vi "Gunner.vi"(8 "error in (no error)":errorcluster, 10 "Map":i32[](array[numeric]), 11 "Gunner In":refnum<class "Cross.lvclass">) -> (0 "error out":errorcluster, 1 "Direction":T1, 2 "Action":T2, 3 "Gunner Out":refnum<class "Cross.lvclass">, 4 "Replicated Class":refnum<class "Cross.lvclass">)   [LabVIEW 2015, in "Cross.lvclass"]
uses:
  Cross.lvclass
  Type Defs/Action Enum.ctl
  Type Defs/Direction Enum.ctl
  Cross.lvclass/Cross.ctl
  Type Defs/SB Type Defs.lvlib
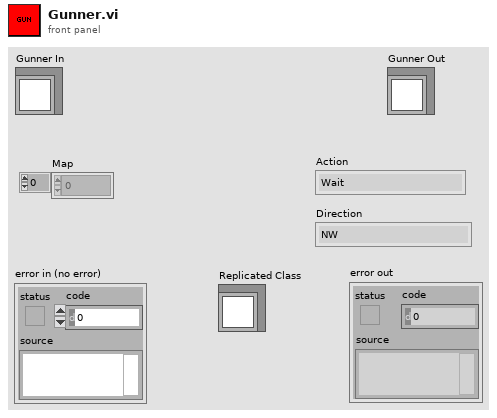
[diagram p1: front panel]
types:
  T1 = typedef "SB Type Defs.lvlib/Direction Enum.ctl" = enum16{"NW", "N", "NE", "E", "SE", "S", "SW", "W"}
  T2 = typedef "SB Type Defs.lvlib/Action Enum.ctl" = enum16{"Wait", "Move", "Attack", "Replicate"}
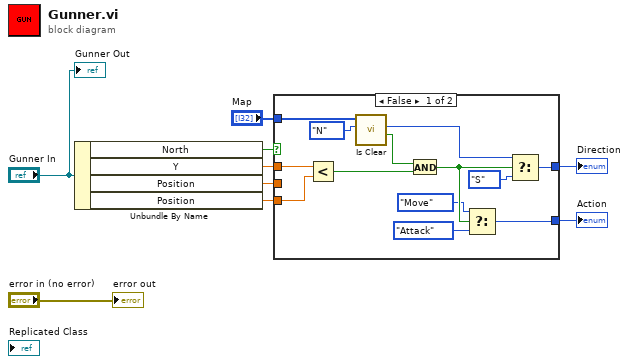
[diagram p0: block diagram]
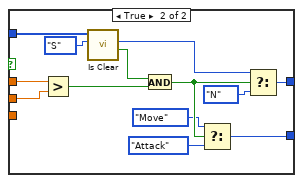
[diagram p2: hidden frame]
diagram:
  n1 = Unbundle By Name("Gunner In") -> ("North"=w7:bool, "Y"=w6:dbl, "Position"=w5:dbl, "Position"=w1:dbl)
  n2 = case shown="False" w7 {
    tunnel: w6 -> [w14 w35]
    tunnel: w5 -> [_ w34]
    tunnel: "Map" -> [w12 w33]
    tunnel: [w10 w24] -> w3
    tunnel: [w11 w23] -> w2
    tunnel: w1 -> [w13 _]
    frame False {
      n3 = Less?(x=w14, y=w13) -> (x < y?=w15:bool)
      n4 = call "Is Clear.vi"("Direction"=Direction_Enum."N", "Maze"=w12) -> ("Can Move?"=w21:bool, "Direction Out"=w19:T1)  [unwired: 6 in, 2 out]
      n5 = And(x=w21, y=w15) -> (x .and. y?=w20:bool)
      n6 = Select(t=Action_Enum."Move" ("Action"), s=w20, f=Action_Enum."Attack" ("Action")) -> (s? t:f=w10:T2)
      n7 = Select(t=w19, s=w20, f=Direction_Enum."S" ("Direction")) -> (s? t:f=w11:T1)
    }
    frame True {
      n8 = Greater?(x=w35, y=w34) -> (0:w30:bool)
      n9 = call "Is Clear.vi"("Direction"=Direction_Enum."S", "Maze"=w33) -> ("Can Move?"=w31:bool, "Direction Out"=w28:T1)  [unwired: 6 in, 2 out]
      n10 = And(x=w31, y=w30) -> (x .and. y?=w29:bool)
      n11 = Select(t=Action_Enum."Move" ("Action"), s=w29, f=Action_Enum."Attack" ("Action")) -> (s? t:f=w24:T2)
      n12 = Select(t=w28, s=w29, f=Direction_Enum."N" ("Direction")) -> (s? t:f=w23:T1)
    }
  }
  "Action" <- w3
  "Direction" <- w2
  "error out" <- "error in (no error)"
  "Gunner Out" <- "Gunner In"
